vi "UPS内部交互全局.vi"() -> ()   [LabVIEW 2016, in "环境动力监测库.lvlib" / "UPS库.lvlib"]
panel:
  out "华为2000-G-UPS参数":T1 {"开机状态" items=["关机", "开机中", "开机失败", "开机完成"]}
  out "华为2000-G-UPS状态":bool[](array[boolean])
  out "华为2000-G-电池状态":T2 {"电池状态" items=["休眠"=2, "浮充"=3, "均充"=4, "放电"=5]}
  out "梦幻城堡C6~20-WA":T3
  out "梦幻城堡C6~20-Q6":T4
  out "通信指示":bool=TRUE
  out "梦幻城堡C1~3Status":T5
  # "输入电压"
  # "输入故障电压"
  # "输出电压"
  # "输出电流百分比"
  # "输入频率"
  # "电池电压"
  # "UPS温度"
  # "UPS状态"
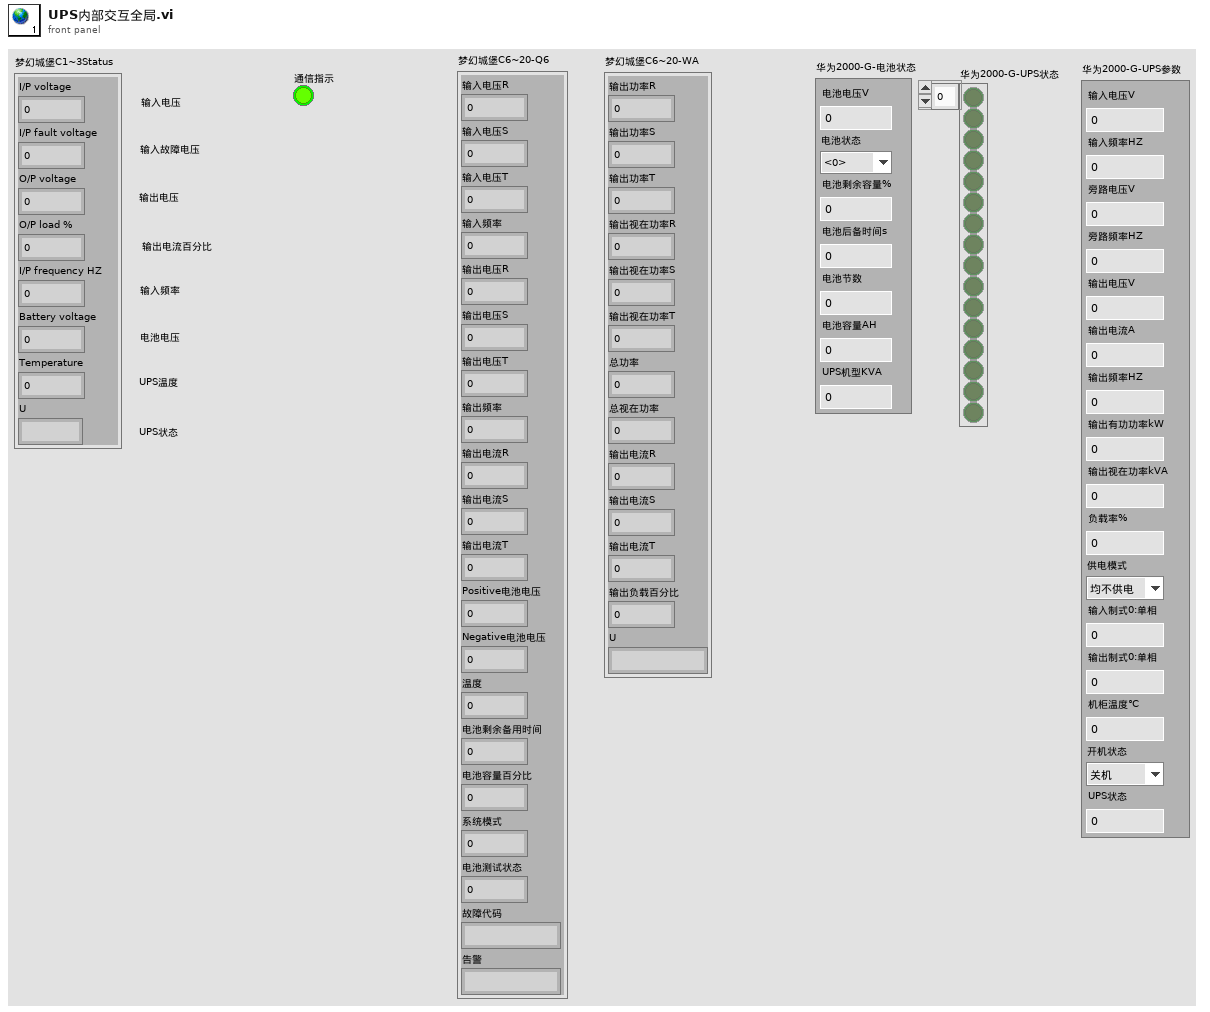
[diagram p1: front panel]
types:
  T1 = cluster{"输入电压V":dbl, "输入频率HZ":dbl, "旁路电压V":dbl, "旁路频率HZ":dbl, "输出电压V":dbl, "输出电流A":dbl, "输出频率HZ":dbl, "输出有功功率kW":dbl, "输出视在功率kVA":dbl, "负载率%":dbl, "供电模式":enum16{"均不供电", "旁路供电", "主路供电", "电池供电", "主路ECO"}, "输入制式0:单相":u16, "输出制式0:单相":u16, "机柜温度℃":dbl, "开机状态":u16, "UPS状态":u8}
  T2 = cluster{"电池电压V":dbl, "电池状态":u16, "电池剩余容量%":u16, "电池后备时间s":u32, "电池节数":u16, "电池容量AH":u16, "UPS机型KVA":u16}
  T3 = cluster{"输出功率R":dbl, "输出功率S":dbl, "输出功率T":dbl, "输出视在功率R":dbl, "输出视在功率S":dbl, "输出视在功率T":dbl, "总功率":dbl, "总视在功率":dbl, "输出电流R":dbl, "输出电流S":dbl, "输出电流T":dbl, "输出负载百分比":dbl, "U":string}
  T4 = cluster{"输入电压R":dbl, "输入电压S":dbl, "输入电压T":dbl, "输入频率":dbl, "输出电压R":dbl, "输出电压S":dbl, "输出电压T":dbl, "输出频率":dbl, "输出电流R":dbl, "输出电流S":dbl, "输出电流T":dbl, "Positive电池电压":dbl, "Negative电池电压":dbl, "温度":dbl, "电池剩余备用时间":dbl, "电池容量百分比":dbl, "系统模式":dbl, "电池测试状态":dbl, "故障代码":string, "告警":string}
  T5 = cluster{"I/P voltage":dbl, "I/P fault voltage":dbl, "O/P voltage":dbl, "O/P load %":dbl, "I/P frequency HZ":dbl, "Battery voltage":dbl, "Temperature":dbl, "U":string}
diagram:
